vi "TEST - Convert Field Value.vi"() -> ()   [LabVIEW 2020, in "InfluxDB v2 Client.lvlib"]
uses:
  InfluxDB v2 Client.lvlib
  Data Type.ctl
panel:
  in  "Boolean":bool
  in  "String":string
  in  "UInteger":u32
  in  "Integer":i32
  out "Field String":string
  in  "Float":dbl format="%.6g"
  out "Variant":variant
  in  "Data Type":T1
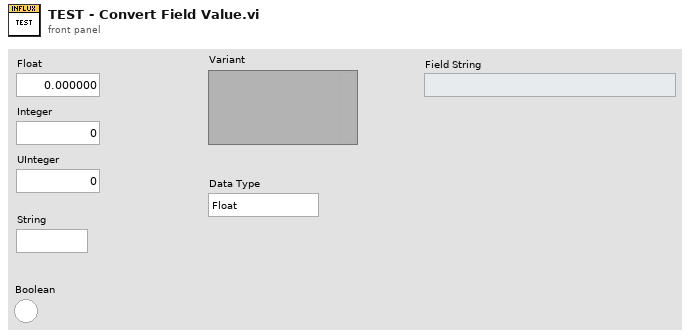
[diagram p1: front panel]
types:
  T1 = typedef "InfluxDB v2 Client.lvlib/Data Type.ctl" = enum16{"Float", "Integer", "UInteger", "String", "Boolean"}
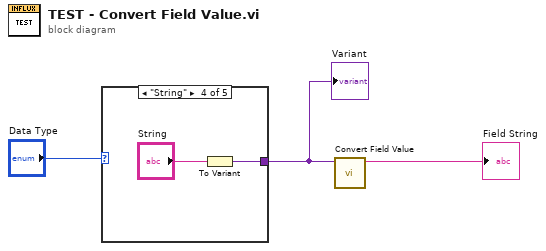
[diagram p0: block diagram]
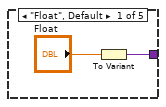
[diagram p2: hidden frame]
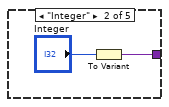
[diagram p3: hidden frame]
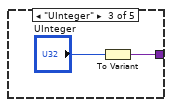
[diagram p4: hidden frame]
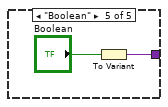
[diagram p5: hidden frame]
diagram:
  n1 = case shown="\"String\"" "Data Type" {
    tunnel: [w4 w7 w9 w11 w13] -> w3
    frame "Float", Default {
      n2 = To Variant(anything="Float") -> (Variant=w4:variant)
    }
    frame "Integer" {
      n3 = To Variant(anything="Integer") -> (Variant=w7:variant)
    }
    frame "UInteger" {
      n4 = To Variant(anything="UInteger") -> (Variant=w9:variant)
    }
    frame "String" {
      n5 = To Variant(anything="String") -> (Variant=w11:variant)
    }
    frame "Boolean" {
      n6 = To Variant(anything="Boolean") -> (Variant=w13:variant)
    }
  }
  "Variant" <- w3
  n7 = call "Convert Field Value.vi"("Field Value"=w3) -> ("Field String"=→"Field String":string)  [unwired: 9 in, 1 out]
